vi "WFGenA02Noise.vi"(1 "Param 0: Frequency":dbl, 2 "Param 1: Inactive":dbl, 3 "Param 2: Inactive":dbl, 4 "Param 3: Inactive":dbl, 5 "error in (no error)":errorcluster, 8 "WFParameters":T2={"Fs (Hz)"=100000.0, "Amp (V)"=5.0, "Ramp (s)"=0.005, "Dur (s)"=0.25} {"Dur (s)" min=0.0 format="%#_4g"; "Ramp (s)" min=0.0; "Fs (Hz)" min=0.0}, 10 "WFRepetitions":T1={"Del (s)"=0.0, "Int (s)"=0.0, "N"=1} {"Int (s)" min=0.0 format="%#_4g"; "Del (s)" min=0.0 format="%#_4f"}) -> (14 "Waveform Out":waveform(dbl)={"t0"=timestamp(0 s since 1904-01-01), "dt"=1e-05, "Y"=array[25000 elements]}, 19 "error out":errorcluster)   [LabVIEW 2013]
uses:
  WFParameters.ctl
  WFRepetitions.ctl
  util/impl/WFComposeA.vi
  <vilib>/measure/NI_MABase.lvlib
panel:
  out "Waveform Graph":waveform(dbl)(graph)={"t0"=timestamp(0 s since 1904-01-01), "dt"=1e-05, "Y"=array[25000 elements]}
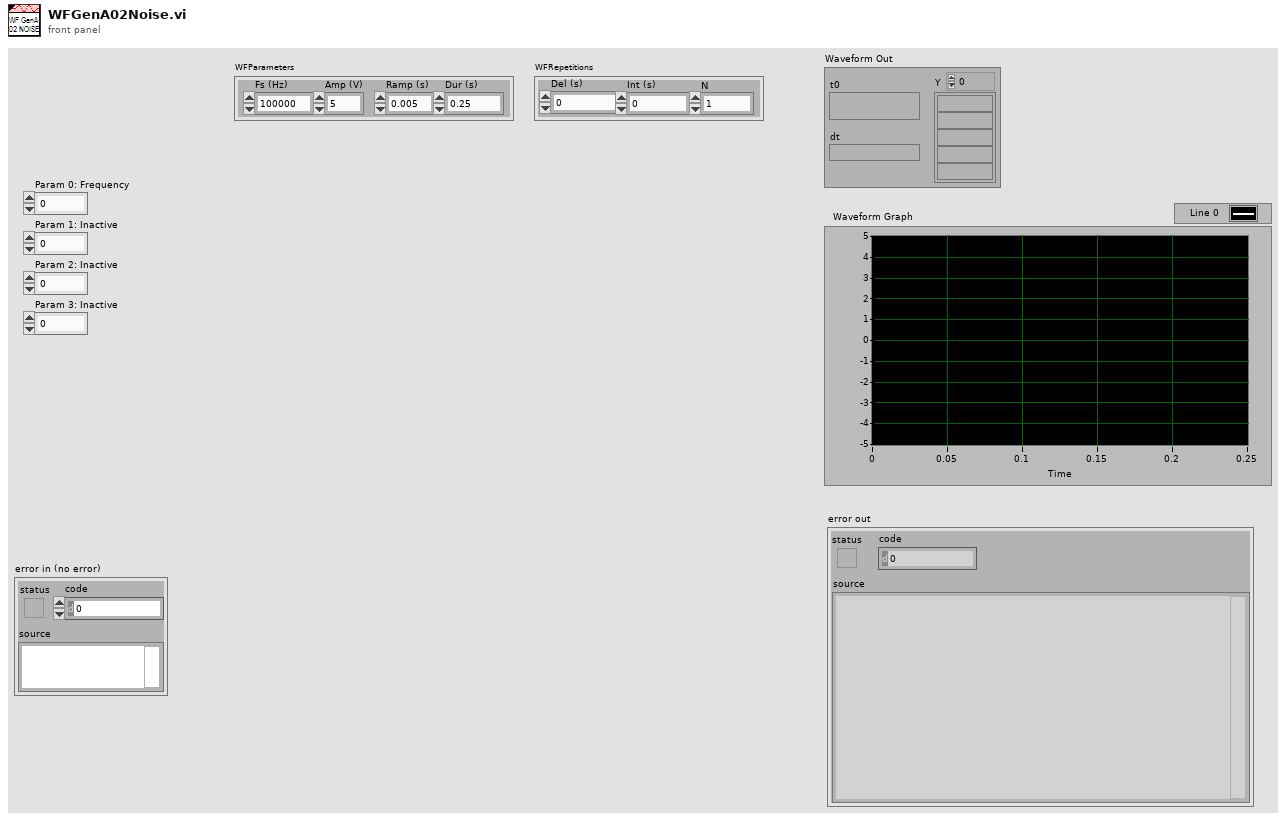
[diagram p1: front panel]
types:
  T1 = typedef "WFRepetitions.ctl" = cluster{"Del (s)":dbl, "Int (s)":dbl, "N":i32}
  T2 = typedef "WFParameters.ctl" = cluster{"Fs (Hz)":dbl, "Amp (V)":dbl, "Ramp (s)":dbl, "Dur (s)":dbl}
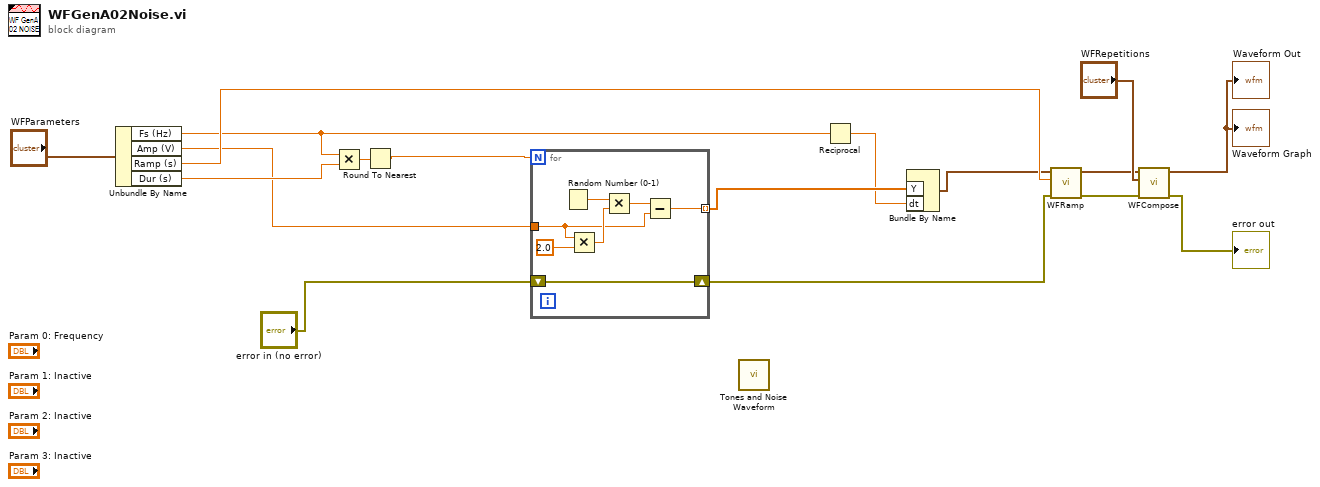
[diagram p0: block diagram]
diagram:
  n1 = Unbundle By Name("WFParameters") -> ("Fs (Hz)"=w3:dbl, "Amp (V)"=w7:dbl, "Ramp (s)"=w9:dbl, "Dur (s)"=w12:dbl)
  n2 = Multiply(x=w3, y=w12) -> (x*y=w13:dbl)
  n3 = Round To Nearest(number=w13) -> (nearest integer value=w8:dbl)
  n4 = for {
    N: w8 -> [_]
    tunnel: w7 -> [w20]
    tunnel: [w19] -> w5 mode=indexing
    shift-right: [w18] -> w2
    shift-left: "error in (no error)" -> [w18]
    n5 = Random Number (0-1)() -> (number: 0 to 1=w24:dbl)
    n6 = Multiply(x=w20, y=2.0) -> (x*y=w22:dbl)
    n7 = Multiply(x=w24, y=w22) -> (x*y=w21:dbl)
    n8 = Subtract(x=w21, y=w20) -> (x-y=w19:dbl)
  }
  n9 = call <vilib>:"Tones and Noise Waveform.vi"() -> ()  [unwired: 10 in, 2 out]
  n10 = Reciprocal(x=w3) -> (1/x=w4:dbl)
  n11 = Bundle By Name("Y"=w5, "dt"=w4) -> (w6:waveform(dbl))  [unwired: 1 in]
  n12 = call "WFRamp.vi"("error in (no error)"=w2, "Ramp Length (s)"=w9, "Waveform In"=w6) -> ("error out"=w10:errorcluster, "Waveform Out"=w11:waveform(dbl))  [unwired: 7 in]
  n13 = call-poly "WFCompose.vi"("error in (no error)"=w10, "WFRepetitions"="WFRepetitions", "Waveform In"=w11) -> ("error out"=→"error out":errorcluster, "Analog Waveform Out"=→"Waveform Graph" →"Waveform Out":waveform(dbl))  [unwired: 7 in]
